vi "1D_Jacobi_eigenvalue_algorithm_v5.vi"() -> ()   [LabVIEW 2020]
uses:
  <vilib>/Analysis/Matrix/Datatypes/RealMatrix.ctl
  <vilib>/Analysis/baseanly.llb/Real A x B.vi
  <vilib>/Analysis/baseanly.llb/Mean (DBL).vi
  <vilib>/Analysis/Matrix/Numeric/Conversions/Array To Matrix - RA2.vi
  <vilib>/Analysis/Matrix/Numeric/Conversions/Matrix To Array - RM.vi
  <vilib>/Analysis/7linalg.llb/Real Eigenvalues and Vectors.vi
  <vilib>/Analysis/Matrix/NI_Matrix.lvlib
  <vilib>/Analysis/NI_AALBase.lvlib
  <vilib>/Analysis/NI_AALPro.lvlib
panel:
  out "A after step #3.3.1 2":sgl[][](array[numeric])
  out "A after step #3.3.1":sgl[][](array[numeric])
  out "A after step #3.2":sgl[][](array[numeric])
  out "A after step #3.1":sgl[][](array[numeric])
  out "index_k_l":i32[](array[numeric])
  out "A[index_k_l]":sgl[](array[numeric])
  out "A[k,l] < abs(A_diff)*1e-36":bool[](array[boolean])
  out "A Diff":sgl[](array[numeric])
  out "t":sgl[](array[numeric])
  out "A after rotation 2":sgl[][](array[numeric])
  out "A after rotation 1":sgl[][](array[numeric])
  out "k":i32[](array[numeric])
  out "l":i32[](array[numeric])
  out "New A[k,k]":sgl
  out "[k,k]":i32
  out "after A[k,k]":sgl[][](array[numeric])
  out "before A[k,k]":sgl[][](array[numeric])
  out "Array 3":bool[][](array[boolean])
  out "Numeric":i32
  out "Array 2":i32[](array[numeric])
  out "Array":i32[](array[numeric])
  out "A after step #2":sgl[][](array[numeric])
  out "Real Matrix":T1
  out "percent error":dbl
  out "FPGA Jacobi eigenvalue":sgl[](array[numeric])
  in  "Number of Rotations":i32=100
  out "A":dbl[][](array[numeric])
  out "LabVIEW eigvals":dbl[](array[numeric])
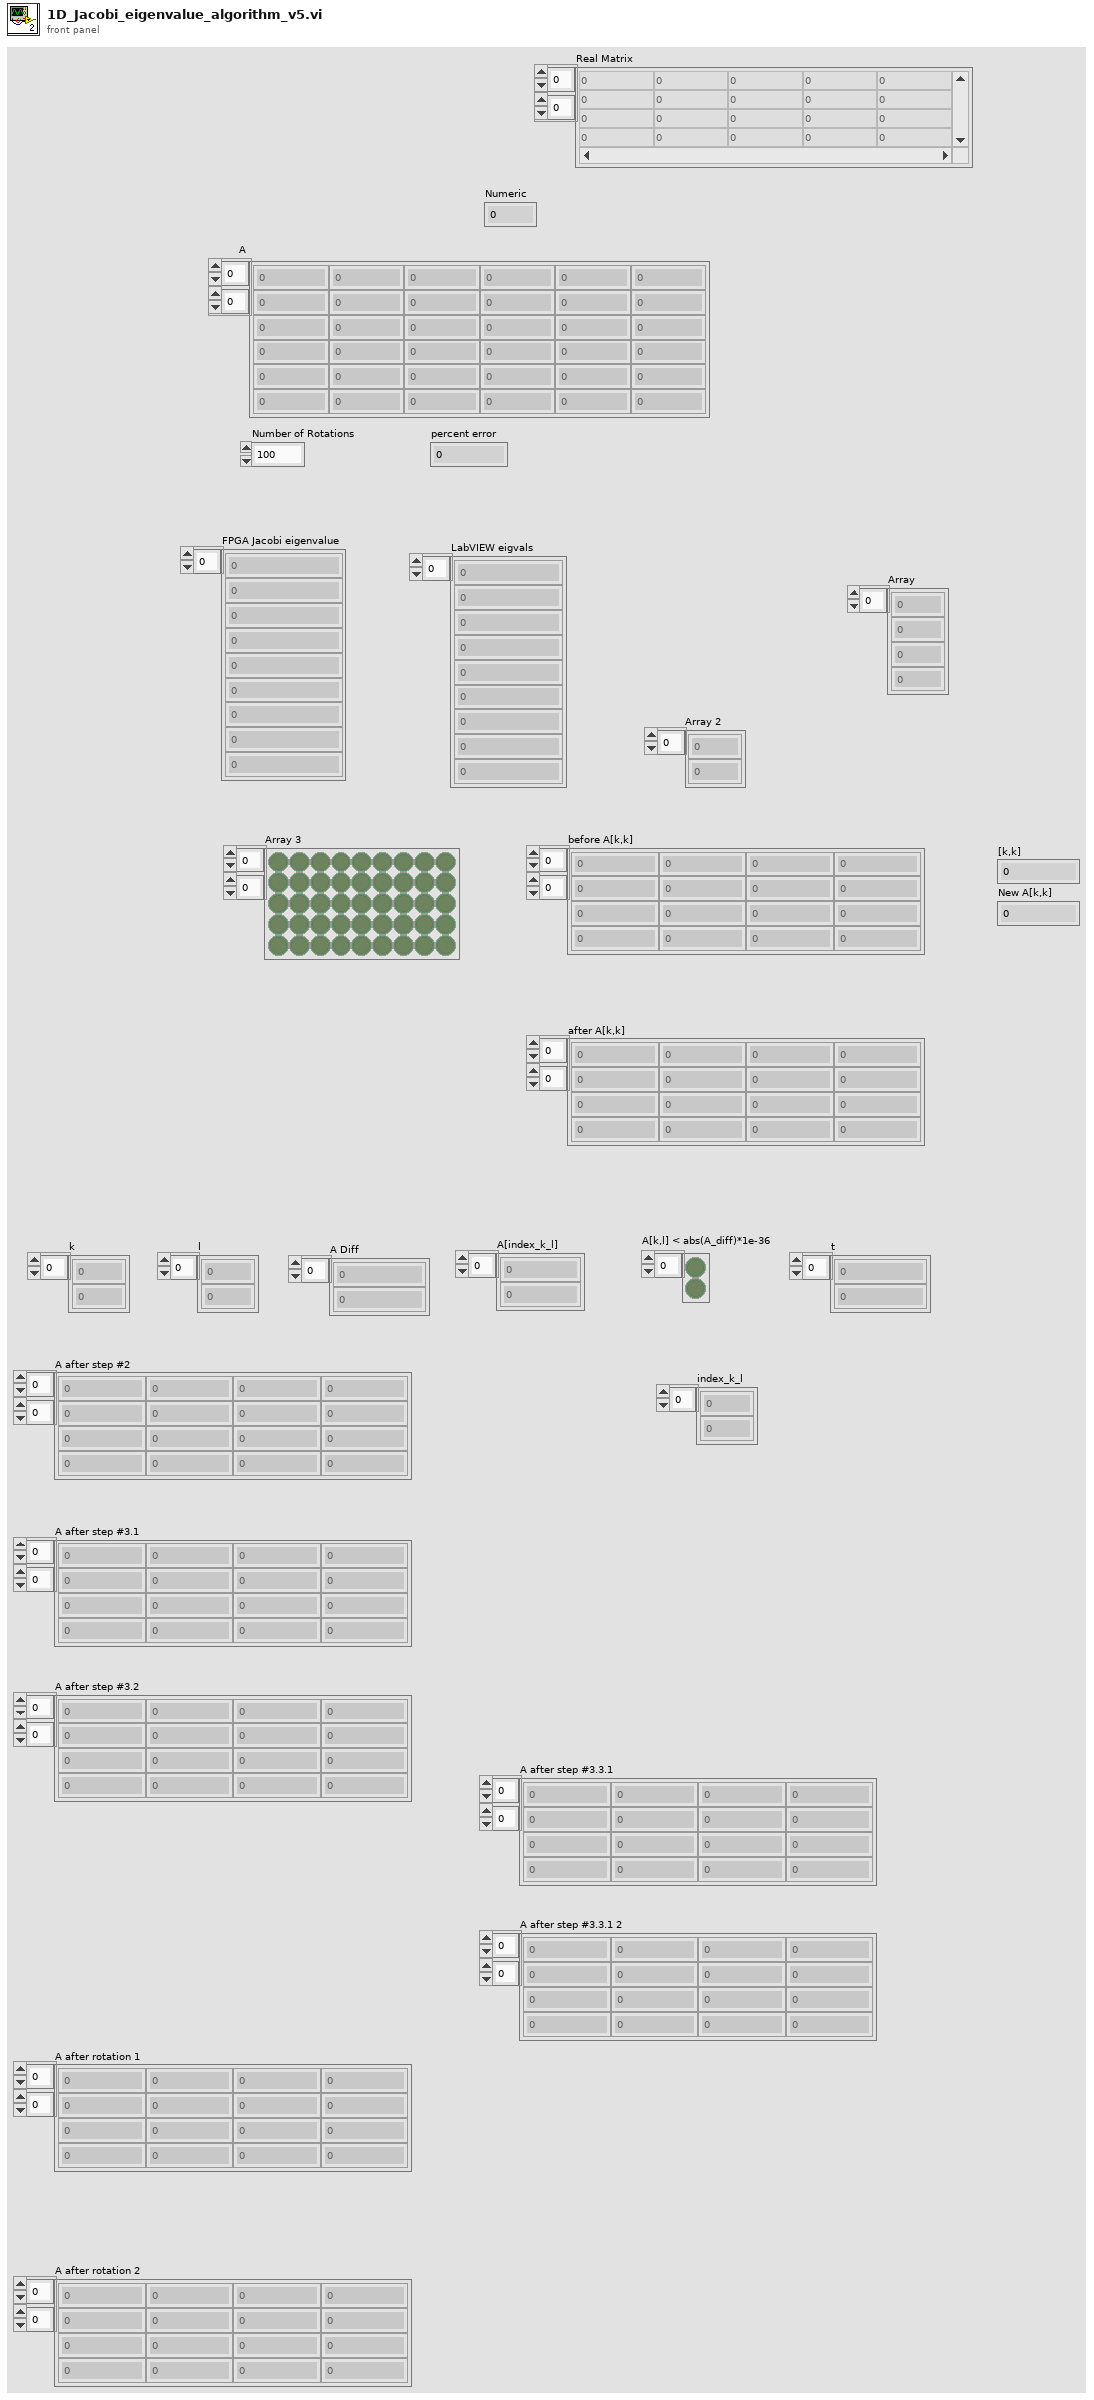
[diagram p1: front panel]
types:
  T1 = typedef "NI_Matrix.lvlib/RealMatrix.ctl" = dbl[][]
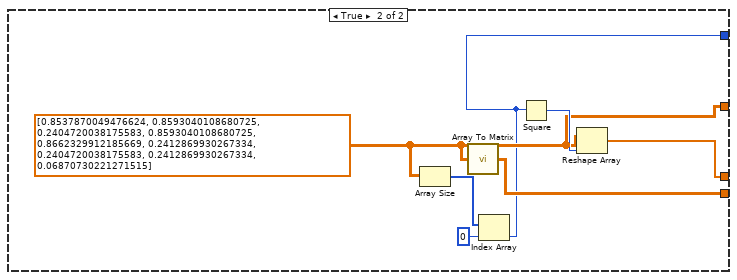
[diagram p3: hidden frame]
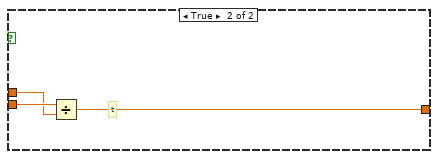
[diagram p5: hidden frame]
diagram:
  w13 = 3 ("dimension size")
  w20 = 3 ("dimension size")
  n1 = case "Use Troubleshooting Matrix" shown="False" FALSE {
    tunnel: [w35 w54] -> w31
    tunnel: [w36 w53] -> w28
    tunnel: [w34 w51] -> w25
    tunnel: [w33 w48] -> w23
    frame False {
      w33 = 30  # n
      n2 = flat-sequence "Make symmetric matrix" {
        tunnel: [w42] -> w35
        tunnel: [w40] -> w36
        tunnel: [w38] -> w34
        tunnel: w33 -> [w37]
        frame #0 {
          n3 = Multiply(x=w37, y=w37) -> (x*y=w39:i32)
          n4 = for {
            N: w39 -> [_]
            tunnel: [w47] -> w46 mode=indexing
            n5 = Random Number (0-1)() -> (number: 0 to 1=w47:dbl)
          }
          n6 = Reshape Array(w46, w37, w37) -> (w45:dbl[][])
          n7 = call-poly <vilib>:"Array To Matrix.vi"("Real 2D Array"=w45) -> ("Real Matrix"=w44:T1)
          n8 = Transpose Matrix(1:w44) -> (0:w43:T1)
          n9 = call-poly <vilib>:"A x B.vi"("B"=w43, "A"=w44) -> ("A x B"=w42:T1)  [unwired: 1 out]
          n10 = call-poly <vilib>:"Matrix To Array.vi"("Real Matrix"=w42) -> ("Real 2D Array"=w38:dbl[][])
          n11 = Reshape Array(w38, w39) -> (w41:dbl[])
          n12 = To Single Precision Float(number=w41) -> (single precision float=w40:sgl[])
        }
      }
    }
    frame True {
      w51 = sgl[][] [[0.853787, 0.859304, 0.240472], [0.859304, 0.866233, 0.241287], [0.240472, 0.241287, 0.0687073]]
      n13 = Array Size(array=w51) -> (size(s)=w50:i32[])
      n14 = call-poly <vilib>:"Array To Matrix.vi"("Real 2D Array"=w51) -> ("Real Matrix"=w54:T1)
      n15 = Index Array(array=w50, index=0) -> (element=w48:i32)
      n16 = Square(x=w48) -> (x^2=w52:i32)
      n17 = Reshape Array(w51, w52) -> (w53:sgl[])
    }
  }
  "A" <- w25
  "Real Matrix" <- w31
  n18 = disable-structure shown="Disabled" {
    frame Disabled {
      (unwired) sgl[][] [[0.414, 0.493, 0.427], [0.493, 0.377, 0.248], [0.427, 0.248, 0.988]]
      # "matrix from python"
    }
    frame Enabled {
    }
  }
  n19 = for "Main Loop: Iterate through each step of the algorithm" {
    N: "Number of Rotations" -> [_]
    tunnel: w23 -> [w99]
    shift-right: [w60] -> w29
    shift-left: w28 -> [w89]
    tunnel: [w62] -> w22 mode=indexing
    tunnel: [w61] -> w21 mode=indexing
    tunnel: [w60] -> w7 mode=indexing
    tunnel: [w59] -> w5 mode=indexing
    tunnel: [w58] -> w4 mode=indexing
    tunnel: [w57] -> w3 mode=indexing
    tunnel: [w56] -> w2 mode=indexing
    tunnel: [w55] -> w1 mode=indexing
    w65 = 3 ("dimension size")
    w68 = 3 ("dimension size")
    (unwired) 0
    w87 = 3 ("dimension size")
    w101 = sgl 0.0  # A max
    # "i_rotation: 0 to number_of_rotations"
    n20 = Decrement(x=w99) -> (x-1=w100:i32)
    n21 = for "Step #1: Find the location (in k,l) in the top triangle with the greatest value" {
      N: w100 -> [_]
      tunnel: w100 -> [w336]
      shift-right: [w340] -> _
      shift-left: w101 -> [w338]
      tunnel: [w339] -> w62
      tunnel: [w337] -> w61
      tunnel: w89 -> [w335]
      tunnel: w99 -> [w334]
      tunnel: [w332] -> w85 mode=indexing
      tunnel: [w331] -> w84 mode=indexing
      i -> [w332]
      # "i_row loop, 0 to (n-1)"
      n22 = Subtract(x=w336, y=w332) -> (x-y=w341:i32)
      n23 = for "For Loop: j" {
        N: w341 -> [_]
        shift-right: [w350] -> w340
        shift-left: w338 -> [w349]
        tunnel: [w342] -> w339
        tunnel: [w346] -> w337
        tunnel: w335 -> [w359]
        tunnel: w332 -> [w348]
        tunnel: w334 -> [w357]
        tunnel: [w353] -> w333 mode=indexing
        tunnel: [w352] -> w331 mode=indexing
        i -> [w353]
        w343 = 0
        # "j_col, 0 to (n-1-i_row)"
        n24 = Compound Arithmetic op=ADD(w353, w348, 1 ("value")) -> (w345:i32)
        n25 = Multiply(x=w357, y=w348) -> (x*y=w355:i32)
        n26 = Add(x=w355, y=w345) -> (x+y=w354:i32)
        n27 = Index Array(array=w359, index=w354) -> (element=w356:sgl)
        n28 = Absolute Value(x=w356) -> (abs(x)=w351:sgl)
        n29 = Greater Or Equal?(x=w351, y=w349) -> (x >= y?=w352:bool)
        n30 = feedback #1(w343) -> (w347:i32)
        n31 = feedback #2(w343) -> (w344:i32)
        n32 = case "if abs(A[i,j+i+1]) >= A_Max:" shown="False" w352 {
          tunnel: [w362 w365] -> w350
          tunnel: w351 -> [_ w365]
          tunnel: w349 -> [w362 _]
          tunnel: w348 -> [_ w364]
          tunnel: [w361 w364] -> w346
          tunnel: w347 -> [w361 _]
          tunnel: w345 -> [_ w363]
          tunnel: [w360 w363] -> w342
          tunnel: w344 -> [w360 _]
          frame False {
          }
          frame True {
          }
        }
        n33 = feedback-in #1(w346) -> ()
        n34 = feedback-in #2(w342) -> ()
      }
      "Array" <- w333
    }
    "Array 2" <- w85
    "Numeric" <- w61
    "Array 3" <- w84
    n35 = flat-sequence "Step #2: Difference of the orthogonal distance & calculate variables for rotation" {
      tunnel: [w109] -> w96
      tunnel: [w108] -> w95
      tunnel: [w107] -> w94
      tunnel: w61 -> [w113]
      tunnel: w99 -> [w112]
      tunnel: w62 -> [w111]
      tunnel: w89 -> [w110]
      tunnel: [w102] -> w81
      tunnel: [w104] -> w80
      tunnel: [w103] -> w77
      tunnel: [w102] -> w55
      tunnel: [w117] -> w93
      tunnel: w96 -> [w119]
      tunnel: w95 -> [w118]
      tunnel: w94 -> [w114]
      tunnel: [w122] -> w82
      tunnel: w81 -> [w122]
      tunnel: w80 -> [w121]
      tunnel: [w121] -> w79
      tunnel: w77 -> [w120]
      tunnel: [w120] -> w76
      tunnel: [w114] -> w74
      tunnel: [w119] -> w72
      tunnel: [w118] -> w70
      tunnel: [w117] -> w59
      tunnel: [w116] -> w58
      tunnel: [w115] -> w57
      tunnel: [w114] -> w56
      tunnel: w93 -> [w155]
      tunnel: [w155] -> w92
      tunnel: [w154] -> w91
      tunnel: [w153] -> w90
      tunnel: [w152] -> w83
      tunnel: w82 -> [w152]
      tunnel: w79 -> [w151]
      tunnel: [w151] -> w78
      tunnel: w76 -> [w150]
      tunnel: [w150] -> w75
      tunnel: w74 -> [w149]
      tunnel: [w149] -> w73
      tunnel: w72 -> [w148]
      tunnel: [w148] -> w71
      tunnel: w70 -> [w147]
      tunnel: [w147] -> w69
      tunnel: [w176] -> w97
      tunnel: [w177] -> w98
      tunnel: w92 -> [w175]
      tunnel: w91 -> [w177]
      tunnel: w90 -> [w176]
      tunnel: w89 -> [w163]
      tunnel: [w164] -> w88
      tunnel: w83 -> [w170]
      tunnel: w78 -> [w169]
      tunnel: w75 -> [w168]
      tunnel: w73 -> [w167]
      tunnel: w71 -> [w166]
      tunnel: w69 -> [w165]
      tunnel: [w162] -> w66
      tunnel: [w161] -> w63
      frame #0 {
        # "Step #2.1: Get K[I,I], K[k,k], K[k,l]"
        n36 = Multiply(x=w111, y=w112) -> (x*y=w106:i32)
        n37 = Multiply(x=w113, y=w112) -> (x*y=w105:i32)
        n38 = Add(x=w106, y=w111) -> (x+y=w103:i32)
        n39 = Add(x=w105, y=w113) -> (x+y=w104:i32)
        n40 = Add(x=w105, y=w111) -> (x+y=w102:i32)
        n41 = Index Array "A[k,k]"(array=w110, index=w104) -> (element=w108:sgl)
        n42 = Index Array "A[l,l]"(array=w110, index=w103) -> (element=w109:sgl)
        n43 = Index Array "A[k,l]"(array=w110, index=w102) -> (element=w107:sgl)
      }
      frame #1 {
        # "Step #2.2: update t or calculate phi and t, A[k,l] < abs(A_diff)*1e-36"
        n44 = Absolute Value(x=w114) -> (abs(x)=w126:sgl)
        n45 = Subtract(x=w119, y=w118) -> (x-y=w116:sgl)
        n46 = Absolute Value(x=w116) -> (abs(x)=w124:sgl)
        n47 = Multiply(x=w124, y=sgl 1e-36 ("x")) -> (x*y=w125:sgl)
        n48 = Less?(x=w126, y=w125) -> (x < y?=w115:bool)
        n49 = case "A[k,l] < abs(A_diff)*1e-36" shown="False" w115 {
          tunnel: w114 -> [w140 w146]
          tunnel: w116 -> [w137 w145]
          tunnel: [w127 w144] -> w117
          frame False {
            n50 = Multiply(x=w140, y=sgl 2.0) -> (x*y=w138:sgl)
            n51 = Divide(x=w137, y=w138) -> (x/y=w131:sgl)
            n52 = Square(x=w131) -> (x^2=w135:sgl)
            n53 = Increment(x=w135) -> (x+1=w134:sgl)
            n54 = Less?(x=w131, y=sgl 0.0) -> (x < y?=w129:bool)
            n55 = Square Root(x=w134) -> (sqrt(x)=w133:sgl)
            n56 = Absolute Value(x=w131) -> (abs(x)=w136:sgl)
            n57 = Add(x=w133, y=w136) -> (x+y=w132:sgl)
            n58 = Reciprocal(x=w132) -> (1/x=w128:sgl)
            n59 = case shown="True" w129 {
              tunnel: w128 -> [w141 w143]
              tunnel: [w141 w142] -> w127
              frame False {
              }
              frame True {
                n60 = Negate(x=w143) -> (-x=w142:sgl)
              }
            }
          }
          frame True {
            # "t"
            n61 = Divide(x=w146, y=w145) -> (x/y=w144:sgl)
          }
        }
      }
      frame #2 {
        # "Step #2.3: Calculate \"tau\""
        n62 = Square(x=w155) -> (x^2=w158:sgl)
        n63 = Increment(x=w158) -> (x+1=w157:sgl)
        n64 = Square Root(x=w157) -> (sqrt(x)=w156:sgl)
        n65 = Reciprocal(x=w156) -> (1/x=w160:sgl)
        n66 = Multiply(x=w160, y=w155) -> (x*y=w154:sgl)
        n67 = Increment(x=w160) -> (x+1=w159:sgl)
        n68 = Divide(x=w154, y=w159) -> (x/y=w153:sgl)
      }
      frame #3 {
        # "Step #2.4: update the A matrix"
        n69 = Multiply(x=w167, y=w175) -> (x*y=w174:sgl)
        n70 = Subtract(x=w165, y=w174) -> (x-y=w172:sgl)
        "New A[k,k]" <- w172
        n71 = Add(x=w166, y=w174) -> (x+y=w171:sgl)
        n72 = Replace Array Subset "A[k,l]"(array=w163, new element=sgl 0.0 ("y"), index=w170) -> (w162:sgl[])
        n73 = Replace Array Subset "A[k,k]"(array=w162, new element=w172, index=w169) -> (w161:sgl[])
        n74 = Replace Array Subset "A[l,l]"(array=w161, new element=w171, index=w168) -> (w164:sgl[])
        "[k,k]" <- w169
      }
    }
    n75 = Reshape Array(w66, w68, w68) -> (→"before A[k,k]":sgl[][])
    n76 = Reshape Array(w63, w65, w65) -> (→"after A[k,k]":sgl[][])
    n77 = Reshape Array(w88, w87, w87) -> (→"A after step #2":sgl[][])
    n78 = flat-sequence "Step #3: Rotate around the high value point" {
      tunnel: w61 -> [w188]
      tunnel: w88 -> [w196]
      tunnel: w99 -> [w189]
      tunnel: w98 -> [w184]
      tunnel: w97 -> [w185]
      tunnel: w62 -> [w187]
      tunnel: [w186] -> w60
      frame #0 {
        w180 = 3 ("dimension size")
        w183 = 3 ("dimension size")
        n79 = for "Step 3.1: Rotate around the high value point" {
          N: w188 -> [_]
          tunnel: w189 -> [w305]
          tunnel: w188 -> [w304]
          tunnel: w184 -> [w299]
          tunnel: w185 -> [w303]
          tunnel: w187 -> [w300]
          shift-right: [w291] -> w182
          shift-left: w196 -> [w298]
          i -> [w306]
          # "i loop, 0 to k"
          n80 = Multiply(x=w305, y=w306) -> (x*y=w301:i32)
          n81 = Add(x=w301, y=w300) -> (x+y=w302:i32)
          n82 = Add(x=w301, y=w304) -> (x+y=w297:i32)
          n83 = flat-sequence "Update A" {
            tunnel: w303 -> [w310]
            tunnel: w302 -> [w311]
            tunnel: w299 -> [w308]
            tunnel: w298 -> [w314]
            tunnel: w297 -> [w309]
            tunnel: [w312] -> w296
            tunnel: [w311] -> w295
            tunnel: [w310] -> w294
            tunnel: [w309] -> w293
            tunnel: [w308] -> w292
            tunnel: [w307] -> w290
            tunnel: w296 -> [w330]
            tunnel: w295 -> [w321]
            tunnel: w294 -> [w329]
            tunnel: w293 -> [w327]
            tunnel: w292 -> [w325]
            tunnel: [w320] -> w291
            tunnel: w290 -> [w319]
            frame #0 {
              # "Step 3.1.1: Update A[i,k]"
              n84 = Index Array "A[i,l]"(array=w314, index=w311) -> (element=w317:sgl)
              n85 = Index Array "A[i,k]"(array=w314, index=w309) -> (element=w307:sgl)
              n86 = Multiply(x=w307, y=w310) -> (x*y=w318:sgl)
              n87 = Add(x=w317, y=w318) -> (x+y=w316:sgl)
              n88 = Multiply(x=w316, y=w308) -> (x*y=w315:sgl)
              n89 = Subtract(x=w307, y=w315) -> (x-y=w313:sgl)
              n90 = Replace Array Subset "A[i,k]"(array=w314, new element=w313, index=w309) -> (w312:sgl[])
            }
            frame #1 {
              # "# Step 3.1.2: Update A[i,l]"
              n91 = Index Array "A[i,k]"(array=w330, index=w327) -> ()  [unwired: 1 out]
              n92 = Index Array "A[i,l]"(array=w330, index=w321) -> (element=w323:sgl)
              n93 = Multiply(x=w323, y=w329) -> (x*y=w328:sgl)
              n94 = Subtract(x=w319, y=w328) -> (x-y=w326:sgl)
              n95 = Multiply(x=w326, y=w325) -> (x*y=w324:sgl)
              n96 = Add(x=w323, y=w324) -> (x+y=w322:sgl)
              n97 = Replace Array Subset "A[i,l]"(array=w330, new element=w322, index=w321) -> (w320:sgl[])
            }
          }
        }
        n98 = Subtract(x=w187, y=1) -> (x-y=w195:i32)
        n99 = Subtract(x=w195, y=w188) -> (x-y=w193:i32)
        n100 = Reshape Array(w182, w183, w183) -> (→"A after step #3.1":sgl[][])
        n101 = for "Step 3.2: Rotate around the high value point" {
          N: w193 -> [_]
          shift-right: [w265] -> w179
          shift-left: w182 -> [w263]
          tunnel: w188 -> [w261]
          tunnel: w189 -> [w257]
          tunnel: w187 -> [w255]
          tunnel: w185 -> [w253]
          tunnel: w184 -> [w251]
          i -> [w260]
          # "i loop, 0 to (l-1-k)"
          n102 = Multiply(x=w261, y=w257) -> (x*y=w259:i32)
          n103 = Compound Arithmetic op=ADD(w260, 1 ("value"), w261) -> (w258:i32)
          n104 = Add(x=w259, y=w258) -> (x+y=w254:i32)
          n105 = Multiply(x=w258, y=w257) -> (x*y=w256:i32)
          n106 = Add(x=w256, y=w255) -> (x+y=w252:i32)
          n107 = flat-sequence "Update A" {
            tunnel: [w277] -> w264
            tunnel: w263 -> [w276]
            tunnel: w254 -> [w268]
            tunnel: w253 -> [w269]
            tunnel: w252 -> [w270]
            tunnel: w251 -> [w267]
            tunnel: [w270] -> w250
            tunnel: [w269] -> w249
            tunnel: [w268] -> w248
            tunnel: [w267] -> w247
            tunnel: [w266] -> w246
            tunnel: [w289] -> w265
            tunnel: w264 -> [w286]
            tunnel: w250 -> [w288]
            tunnel: w249 -> [w287]
            tunnel: w248 -> [w285]
            tunnel: w247 -> [w282]
            tunnel: w246 -> [w278]
            frame #0 {
              # "Step 3.2.1: Update A[k,i+1+k]"
              n108 = Index Array "A[i+1+k,l?]"(array=w276, index=w270) -> (element=w275:sgl)
              n109 = Index Array "A[k,i+1+k?]"(array=w276, index=w268) -> (element=w266:sgl)
              n110 = Multiply(x=w266, y=w269) -> (x*y=w274:sgl)
              n111 = Add(x=w275, y=w274) -> (x+y=w273:sgl)
              n112 = Multiply(x=w273, y=w267) -> (x*y=w272:sgl)
              n113 = Subtract(x=w266, y=w272) -> (x-y=w271:sgl)
              n114 = Replace Array Subset "A[k,i+1+k?]"(array=w276, new element=w271, index=w268) -> (w277:sgl[])
            }
            frame #1 {
              # "Step 3.2.2: Update A[i+1+k,l]"
              n115 = Index Array "A[i+1+k,l?]"(array=w286, index=w288) -> (element=w280:sgl)
              n116 = Multiply(x=w280, y=w287) -> (x*y=w284:sgl)
              n117 = Index Array "A[k,i+1+k]"(array=w286, index=w285) -> ()  [unwired: 1 out]
              n118 = Subtract(x=w278, y=w284) -> (x-y=w283:sgl)
              n119 = Multiply(x=w283, y=w282) -> (x*y=w281:sgl)
              n120 = Add(x=w280, y=w281) -> (x+y=w279:sgl)
              n121 = Replace Array Subset "A[i+1+k,l?]"(array=w286, new element=w279, index=w288) -> (w289:sgl[])
            }
          }
        }
        n122 = Subtract(x=w189, y=1) -> (x-y=w191:i32)
        n123 = Subtract(x=w191, y=w187) -> (x-y=w190:i32)
        n124 = Reshape Array(w179, w180, w180) -> (→"A after step #3.2":sgl[][])
        n125 = for "Step 3.3: Rotate around the high value point" {
          N: w190 -> [_]
          tunnel: w189 -> [w217]
          tunnel: w188 -> [w221]
          tunnel: w187 -> [w216]
          shift-right: [w198] -> w186
          shift-left: w179 -> [w212]
          tunnel: w185 -> [w210]
          tunnel: w184 -> [w208]
          i -> [w220]
          w200 = 3 ("dimension size")
          w203 = 3 ("dimension size")
          # "i loop, 0 to (n-1-l)"
          n126 = Multiply(x=w217, y=w216) -> (x*y=w215:i32)
          n127 = Multiply(x=w221, y=w217) -> (x*y=w218:i32)
          n128 = Compound Arithmetic op=ADD(w220, 1 ("value"), w216) -> (w214:i32)
          n129 = Add(x=w215, y=w214) -> (x+y=w209:i32)
          n130 = Add(x=w218, y=w214) -> (x+y=w211:i32)
          n131 = flat-sequence "Update A" {
            tunnel: [w223] -> w213
            tunnel: w212 -> [w229]
            tunnel: w211 -> [w225]
            tunnel: w210 -> [w226]
            tunnel: w209 -> [w227]
            tunnel: w208 -> [w224]
            tunnel: [w227] -> w207
            tunnel: [w226] -> w206
            tunnel: [w225] -> w205
            tunnel: [w224] -> w204
            tunnel: [w223] -> w202
            tunnel: [w222] -> w197
            tunnel: [w245] -> w198
            tunnel: w213 -> [w242]
            tunnel: w207 -> [w244]
            tunnel: w206 -> [w243]
            tunnel: w205 -> [w241]
            tunnel: w204 -> [w238]
            tunnel: w197 -> [w234]
            frame #0 {
              # "Step 3.3.1: Update A[k,i+1+l]"
              n132 = Index Array "A[k,i+1+l]"(array=w229, index=w225) -> (element=w222:sgl)
              n133 = Index Array "A[l,i+1+l]"(array=w229, index=w227) -> (element=w232:sgl)
              n134 = Multiply(x=w222, y=w226) -> (x*y=w233:sgl)
              n135 = Add(x=w233, y=w232) -> (x+y=w231:sgl)
              n136 = Multiply(x=w231, y=w224) -> (x*y=w230:sgl)
              n137 = Subtract(x=w222, y=w230) -> (x-y=w228:sgl)
              n138 = Replace Array Subset "A[i+1+k,l]"(array=w229, new element=w228, index=w225) -> (w223:sgl[])
            }
            frame #1 {
              # "Step 3.3.2: Update A[l,i+1+l]"
              n139 = Index Array "A[k,i+1+l]"(array=w242, index=w241) -> ()  [unwired: 1 out]
              n140 = Index Array "A[l,i+1+l]"(array=w242, index=w244) -> (element=w236:sgl)
              n141 = Multiply(x=w236, y=w243) -> (x*y=w240:sgl)
              n142 = Subtract(x=w234, y=w240) -> (x-y=w239:sgl)
              n143 = Multiply(x=w239, y=w238) -> (x*y=w237:sgl)
              n144 = Add(x=w237, y=w236) -> (x+y=w235:sgl)
              n145 = Replace Array Subset "A[l,i_1+l]"(array=w242, new element=w235, index=w244) -> (w245:sgl[])
            }
          }
          n146 = Reshape Array(w202, w203, w203) -> (→"A after step #3.3.1":sgl[][])
          n147 = Reshape Array(w198, w200, w200) -> (→"A after step #3.3.1 2":sgl[][])
        }
      }
    }
  }
  "l" <- w22
  "k" <- w21
  "t" <- w5
  "A Diff" <- w4
  "A[k,l] < abs(A_diff)*1e-36" <- w3
  "A[index_k_l]" <- w2
  "index_k_l" <- w1
  n148 = call-poly <vilib>:"Eigenvalues and Vectors.vi"("Input Matrix"=w31) -> ("Eigenvalues"=w32:cdb[])  [unwired: 2 in, 2 out]
  n149 = Complex To Re/Im(x + iy=w32) -> (x=w26:dbl[])  [unwired: 1 out]
  n150 = Array Subset(array=w7, index (row)=0 ("index"), length (row)=1 ("length"), index (col)=0 ("index"), length (col)=9 ("length")) -> (w17:sgl[][])
  n151 = Reshape Array(w17, w20, w20) -> (→"A after rotation 1":sgl[][])
  n152 = flat-sequence "Step 4: extract the Eigen values from the diagonal" {
    tunnel: w29 -> [w368]
    tunnel: w23 -> [w367]
    tunnel: [w366] -> w27
    frame #0 {
      n153 = for "Eigenvalue vector" {
        N: w367 -> [_]
        tunnel: [sgl 0.0] -> w369 mode=indexing
      }
      n154 = for "Eigenvalue vector" {
        N: w367 -> [_]
        shift-right: [w376] -> w366
        shift-left: w369 -> [w377]
        tunnel: w368 -> [w375]
        tunnel: w367 -> [w374]
        i -> [w372]
        n155 = Multiply(x=w374, y=w372) -> (x*y=w373:i32)
        n156 = Add(x=w373, y=w372) -> (x+y=w371:i32)
        n157 = Index Array "A[k,i+1+l?]"(array=w375, index=w371) -> (element=w370:sgl)
        n158 = Replace Array Subset(array=w377, new element=w370, index=w372) -> (w376:sgl[])
      }
    }
  }
  n159 = Array Subset(array=w7, index (row)=1 ("index"), length (row)=1 ("length"), index (col)=0 ("index"), length (col)=9 ("length")) -> (w11:sgl[][])
  n160 = Reshape Array(w11, w13, w13) -> (→"A after rotation 2":sgl[][])
  n161 = flat-sequence "Calculate the percent error" {
    tunnel: w27 -> [w390]
    tunnel: w26 -> [w389]
    frame #0 {
      n162 = Sort 1D Array(array=w389) -> (sorted array=w388:dbl[])
      "LabVIEW eigvals" <- w388
      n163 = Sort 1D Array(array=w390) -> (sorted array=w387:sgl[])
      "FPGA Jacobi eigenvalue" <- w387
      n164 = To Single Precision Float(number=w388) -> (single precision float=w384:sgl[])
      n165 = Subtract(x=w387, y=w384) -> (x-y=w386:sgl[])
      n166 = Absolute Value(x=w386) -> (abs(x)=w385:sgl[])
      n167 = Divide(x=w385, y=w384) -> (x/y=w383:sgl[])
      n168 = Absolute Value(x=w383) -> (abs(x)=w382:sgl[])
      n169 = call-poly <vilib>:"Mean.vi"("X"=w382) -> ("mean"=w381:dbl)  [unwired: 1 out]
      n170 = Multiply(x=w381, y=100.0) -> (x*y=→"percent error":dbl)
    }
  }
